vi "NewGame.vi"(7 "BouncerType (ChildObject)":refnum<class "Bouncer.lvclass">, 8 "error in (no error)":errorcluster, 11 "FPGA_ref":T1) -> (0 "error out":errorcluster, 3 "Bouncer out":refnum<class "Bouncer.lvclass">)   [LabVIEW 2019, in "RT_Game.lvlib" / "Bouncer.lvclass"]
uses:
  Bouncer.lvclass
  C:/Users/FreshBob/Dropbox/VIs/myRIO_GameConsole/RT/RT_Game/Game/Game.lvclass
  FPGA_Interface.ctl
  PongBall/PongBall.lvclass
  C:/Users/FreshBob/Dropbox/VIs/myRIO_GameConsole/RT/RT_Game/GameObject/GameObject.lvclass
  PongPanel/PongPanel.lvclass
  C:/Users/FreshBob/Dropbox/VIs/myRIO_GameConsole/RT/RT_Game/RT_Sprite/RT_Sprite.lvclass
  Game/Coordinate.ctl
  Bouncer.lvclass/Bouncer.ctl
  PongBall/PongBall.lvclass/PongBall.ctl
  GameObject/GameObject.lvclass/GameObject.ctl
  PongPanel/PongPanel.lvclass/PongPanel.ctl
  PongBall/Write start_pos.vi
  GameObject/Write friction.vi
  GameObject/Write Damping.vi
  GameObject/Write MaxSpeed.vi
  GameObject/Write MinSpeed.vi
  GameObject/Write MaxSpeedX.vi
  GameObject/Write MinSpeedX.vi
  GameObject/Read Velocity.vi
  GameObject/Write Velocity.vi
  PongPanel/Write StartPos.vi
  PongPanel/Write limit_y.vi
  PongPanel/Write limit_y_down.vi
  PongPanel/Write Speed.vi
  PongPanel/Write limit_x_down.vi
  PongPanel/Write limit_x_up.vi
  GameObject/Write IsActive.vi
  Game/Game.lvclass
  RT_Sprite/RT_Sprite.lvclass
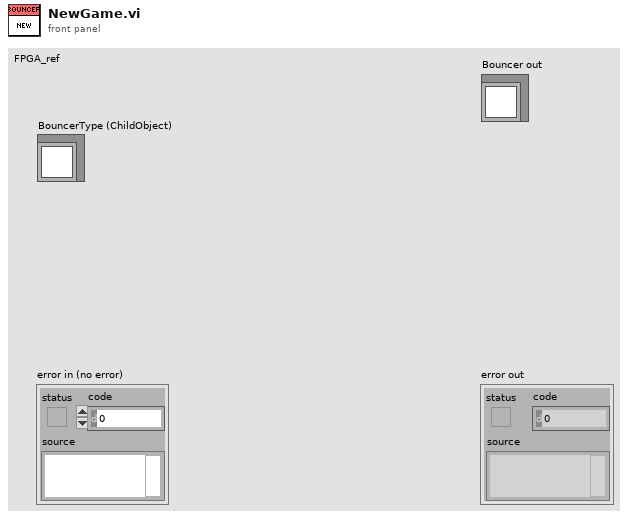
[diagram p1: front panel]
types:
  T1 = typedef "FPGA_Interface.ctl" = refnum<k20>
  T2 = enum16{"all", "up", "down", "left", "right", "leftup", "rightup", "leftdown", "rightdown"}
  T3 = typedef "RT_Game.lvlib/Game.lvclass/Coordinate.ctl" = cluster{"x":dbl, "y":dbl}
  T4 = typedef "RT_Game.lvlib/Velocity.ctl" = cluster{"x":dbl, "y":dbl}
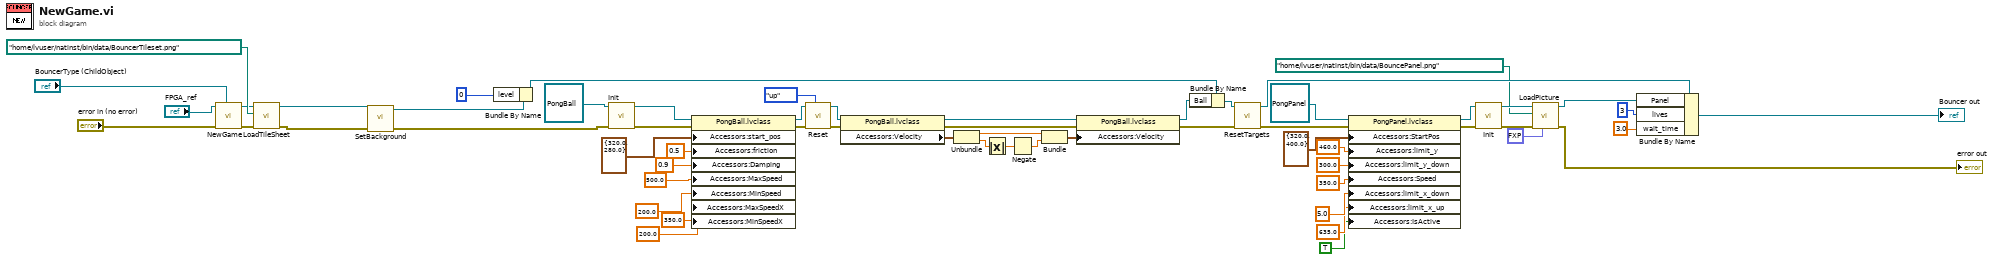
[diagram p0: block diagram]
diagram:
  n1 = call-parent "NewGame.vi"("GameType (ChildObject)"="BouncerType (ChildObject)", "error in (no error)"="error in (no error)", "FPGA_ref"="FPGA_ref") -> ("error out"=w59:errorcluster, "Game out"=w2:refnum<class "Bouncer.lvclass">)  [unwired: 7 in]
  n2 = call "LoadTileSheet.vi"("error in (no error)"=w59, "Tile Path"=path "/home/lvuser/natinst/bin/data/BouncerTileset.png", "Game in"=w2) -> ("error out"=w34:errorcluster, "Game out"=w1:refnum<class "Bouncer.lvclass">)  [unwired: 7 in]
  n3 = call "SetBackground.vi"("error in (no error)"=w34, "Bouncer in"=w1) -> ("error out"=w32:errorcluster, "Bouncer out"=w31:refnum<class "Bouncer.lvclass">)  [unwired: 8 in]
  n4 = Bundle By Name(cluster=w31, "level"=i16 0) -> (w12:refnum<class "Bouncer.lvclass">)
  n5 = call-dynamic "Init.vi"("error in (no error)"=w32, "PongBall in"=refnum<class "PongBall.lvclass"> refnum ("Ball")) -> ("error out"=w54:errorcluster, "PongBall out"=w19:refnum<class "PongBall.lvclass">)  [unwired: 8 in]
  n6 = property class="PongBall.lvclass"(reference=w19, error in=w54, "Accessors:start_pos"=T3 {"x"=320.0, "y"=280.0} ("start_pos"), "Accessors:friction"=0.5 ("friction"), "Accessors:Damping"=0.9 ("Damping"), "Accessors:MaxSpeed"=500.0 ("MaxSpeed"), "Accessors:MinSpeed"=200.0 ("MinSpeed"), "Accessors:MaxSpeedX"=350.0 ("MaxSpeedX"), "Accessors:MinSpeedX"=200.0 ("MinSpeedX")) -> (reference out=w16:refnum<class "PongBall.lvclass">, error out=w20:errorcluster)
  n7 = call "Reset.vi"("Direction (all)"=T2."up", "error in (no error)"=w20, "PongBall in"=w16) -> ("error out"=w17:errorcluster, "PongBall out"=w15:refnum<class "PongBall.lvclass">)  [unwired: 7 in]
  n8 = property class="PongBall.lvclass"(reference=w15, error in=w17) -> (reference out=w27:refnum<class "PongBall.lvclass">, error out=w28:errorcluster, "Accessors:Velocity"=w26:T4)
  n9 = Unbundle(w26) -> ("x"=w25:dbl, "y"=w24:dbl)
  n10 = Absolute Value(x=w24) -> (abs(x)=w23:dbl)
  n11 = Negate(x=w23) -> (-x=w22:dbl)
  n12 = Bundle("x"=w25, w22) -> (w21:cluster{"x":dbl, dbl})  [unwired: 1 in]
  n13 = property class="PongBall.lvclass"(reference=w27, error in=w28, "Accessors:Velocity"=w21) -> (reference out=w29:refnum<class "PongBall.lvclass">, error out=w30:errorcluster)
  n14 = Bundle By Name(cluster=w12, "Ball"=w29) -> (w51:refnum<class "Bouncer.lvclass">)
  n15 = call "ResetTargets.vi"("error in (no error)"=w30, "Bouncer in"=w51) -> ("error out"=w53:errorcluster, "Bouncer out"=w52:refnum<class "Bouncer.lvclass">)  [unwired: 8 in]
  n16 = property class="PongPanel.lvclass"(reference=refnum<class "PongPanel.lvclass"> refnum ("RT_Game.lvlib:PongPanel.lvclass"), error in=w53, "Accessors:StartPos"=T3 {"x"=320.0, "y"=400.0} ("StartPos"), "Accessors:limit_y"=460.0 ("limit_y"), "Accessors:limit_y_down"=300.0 ("limit_y_down"), "Accessors:Speed"=350.0 ("Speed"), "Accessors:limit_x_down"=5.0 ("limit_x_down"), "Accessors:limit_x_up"=635.0 ("limit_x_up"), "Accessors:IsActive"=TRUE ("IsActive")) -> (reference out=w47:refnum<class "PongPanel.lvclass">, error out=w49:errorcluster)
  n17 = call-dynamic "Init.vi"("error in (no error)"=w49, "PongPanel in"=w47) -> ("error out"=w50:errorcluster, "PongPanel out"=w39:refnum<class "PongPanel.lvclass">)  [unwired: 8 in]
  n18 = call "LoadPicture.vi"("Transparent Color"=fxp<+,3,3> 4.0, "error in (no error)"=w50, "Picture Path"=path "/home/lvuser/natinst/bin/data/BouncePanel.png", "RT_Sprite in"=w39) -> ("error out"=→"error out":errorcluster, "RT_Sprite out"=w36:refnum<class "PongPanel.lvclass">)  [unwired: 6 in]
  n19 = Bundle By Name(cluster=w52, "Panel"=w36, "lives"=i16 3, "wait_time"=3.0) -> (→"Bouncer out":refnum<class "Bouncer.lvclass">)
